vi "Set_Asc.vi"(1 "timeOfExposure (32 bit)":u32=5000, 2 "numOfScans":u16=4) -> ()   [LabVIEW 2012]
uses:
  hidapi_32bits.dll
panel:
  out "flag get Acq param":i32
  out "flag get frame format":i32
  out "flag Set Acq param":i32
  out "flag_setFrame":i32
  in  "timeOfExposure":u32
  in  "scanMode":u8
  in  "numOfBlankScans":u16
  in  "numOfScans":u16
  in  "numOfPixelsInFrame":u16
  in  "numOfPixelsInFrame":u16
  in  "reductionMode":u8
  in  "numOfEndElement":u16
  in  "numOfStartElement":u16
  in  "scanMode":u8=3
  in  "numOfBlankScans":u16
  in  "reductionMode":u8
  in  "numOfEndElement":u16=3647
  in  "numOfStartElement":u16
  # "(averaging)"
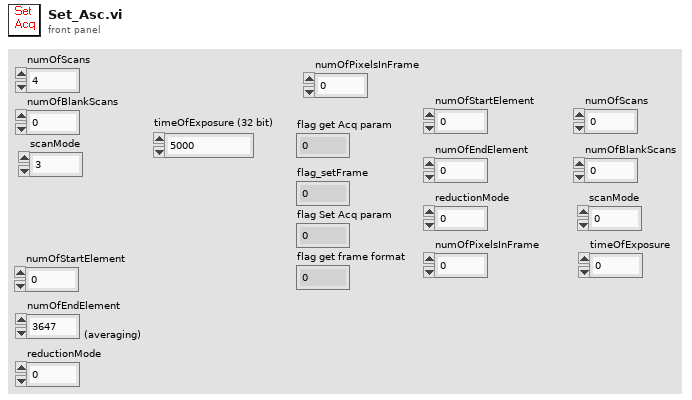
[diagram p1: front panel]
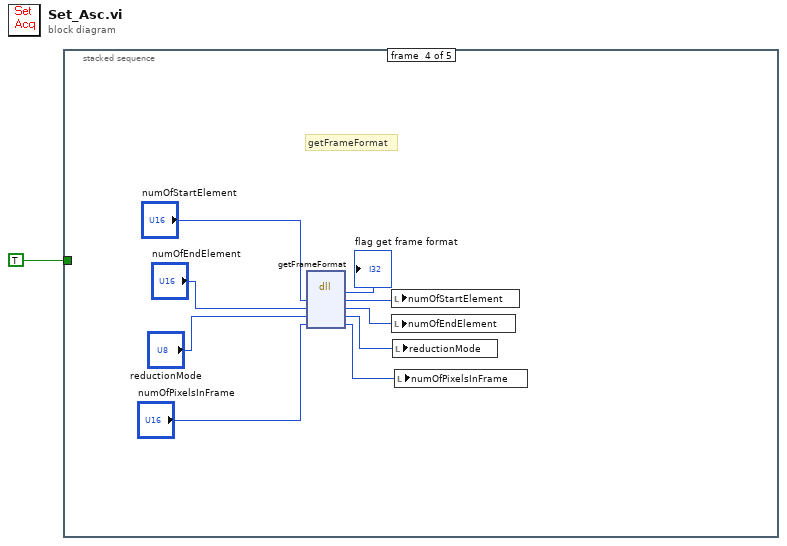
[diagram p0: block diagram]
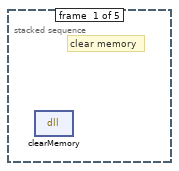
[diagram p2: hidden frame]
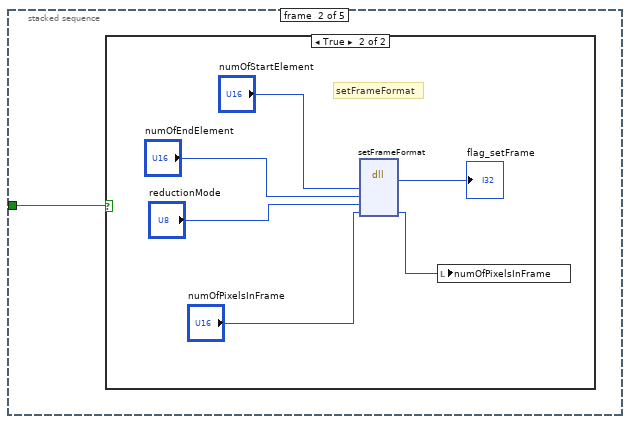
[diagram p3: hidden frame]
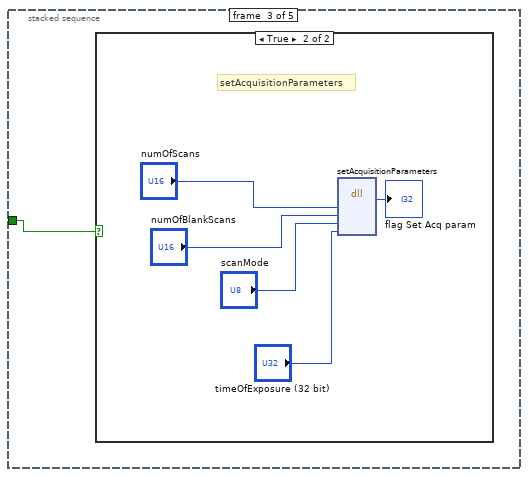
[diagram p5: hidden frame]
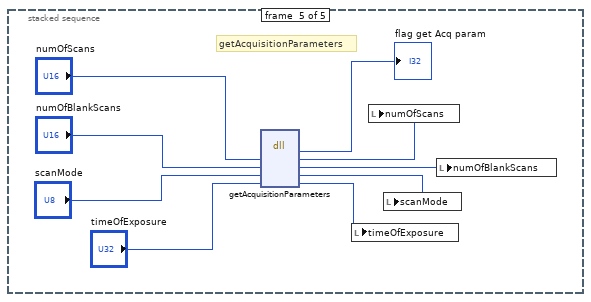
[diagram p7: hidden frame]
diagram:
  n1 = stacked-sequence {
    tunnel: TRUE -> [_ w2 w9 _ _]
    frame #0 {
      # "clear memory"
      n2 = dll-call lib="C:/All_Data/mikrocont/Project1/New_controller__Jan_2015/LabView_Aug_2015/hidapi_32bits.dll" fn="clearMemory"() -> ()  [unwired: 4 in, 2 out]
    }
    frame #1 {
      n3 = case shown="True" w2 {
        frame False {
        }
        frame True {
          # "setFrameFormat"
          n4 = dll-call lib="C:/All_Data/mikrocont/Project1/New_controller__Jan_2015/LabView_Aug_2015/hidapi_32bits.dll" fn="setFrameFormat"("numOfStartElement"="numOfStartElement", "numOfEndElement"="numOfEndElement", "reductionMode"="reductionMode", "numOfPixelsInFrame"="numOfPixelsInFrame") -> ("return type"=→"flag_setFrame":i32, "numOfPixelsInFrame"=w4:u16)  [unwired: 6 in, 2 out]
          n5 = local write "numOfPixelsInFrame"(w4) -> ()
        }
      }
    }
    frame #2 {
      n6 = case shown="True" w9 {
        frame False {
        }
        frame True {
          # "setAcquisitionParameters"
          n7 = dll-call lib="C:/All_Data/mikrocont/Project1/New_controller__Jan_2015/LabView_Aug_2015/hidapi_32bits.dll" fn="setAcquisitionParameters"("numOfScans"="numOfScans", "numOfBlankScans"="numOfBlankScans", "scanMode"="scanMode", "exposureTime"="timeOfExposure (32 bit)") -> ("return type"=→"flag Set Acq param":i32)  [unwired: 7 in, 2 out]
        }
      }
    }
    frame #3 {
      # "getFrameFormat"
      n8 = dll-call lib="C:/All_Data/mikrocont/Project1/New_controller__Jan_2015/LabView_Aug_2015/hidapi_32bits.dll" fn="getFrameFormat"("numOfStartElement"="numOfStartElement", "numOfEndElement"="numOfEndElement", "reductionMode"="reductionMode", "numOfPixelsInFrame"="numOfPixelsInFrame") -> ("return type"=→"flag get frame format":i32, "numOfStartElement"=w19:u16, "numOfEndElement"=w18:u16, "reductionMode"=w17:u8, "numOfPixelsInFrame"=w16:u16)  [unwired: 3 in, 2 out]
      n9 = local write "numOfStartElement"(w19) -> ()
      n10 = local write "numOfEndElement"(w18) -> ()
      n11 = local write "reductionMode"(w17) -> ()
      n12 = local write "numOfPixelsInFrame"(w16) -> ()
    }
    frame #4 {
      # "getAcquisitionParameters"
      n13 = dll-call lib="C:/All_Data/mikrocont/Project1/New_controller__Jan_2015/LabView_Aug_2015/hidapi_32bits.dll" fn="getAcquisitionParameters"("numOfScans"="numOfScans", "numOfBlankScans"="numOfBlankScans", "scanMode"="scanMode", "timeOfExposure"="timeOfExposure") -> ("return type"=→"flag get Acq param":i32, "numOfScans"=w31:u16, "numOfBlankScans"=w29:u16, "scanMode"=w27:u8, "timeOfExposure"=w25:u32)  [unwired: 3 in, 2 out]
      n14 = local write "timeOfExposure"(w25) -> ()
      n15 = local write "numOfScans"(w31) -> ()
      n16 = local write "scanMode"(w27) -> ()
      n17 = local write "numOfBlankScans"(w29) -> ()
    }
  }
